vi "string H.vi"() -> ()   [LabVIEW 2020]
panel:
  out "data string":string
  out "*(type *) &x":string
  in  "Numeric":i16
  out "match substring 2":string
  out "before substring 2":string
  out "match substring":string
  out "before substring":string
  out "result string":string
  in  "number":dbl
  in  "age":dbl
  in  "name":string
  out "trimmed length":i32
  out "trimmed string":string
  out "String Subset":string
  out "length":i32
  out "concatonated":string
  in  "String":string
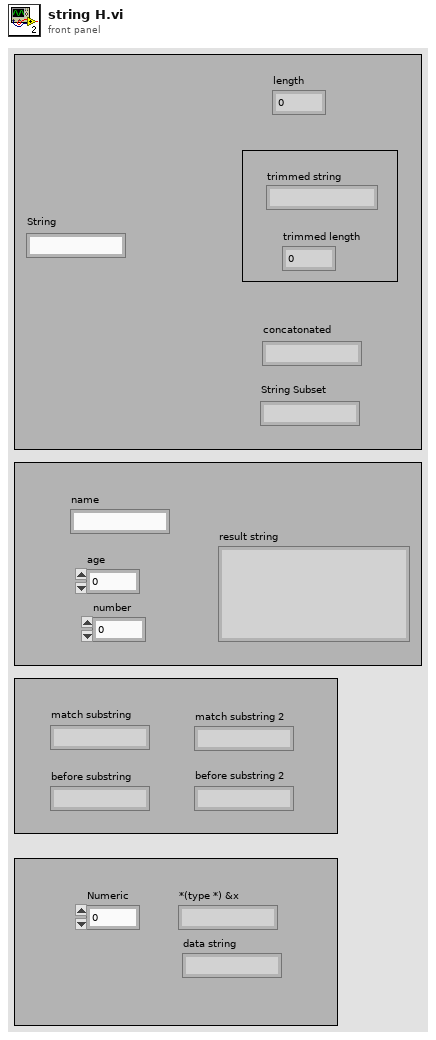
[diagram p1: front panel]
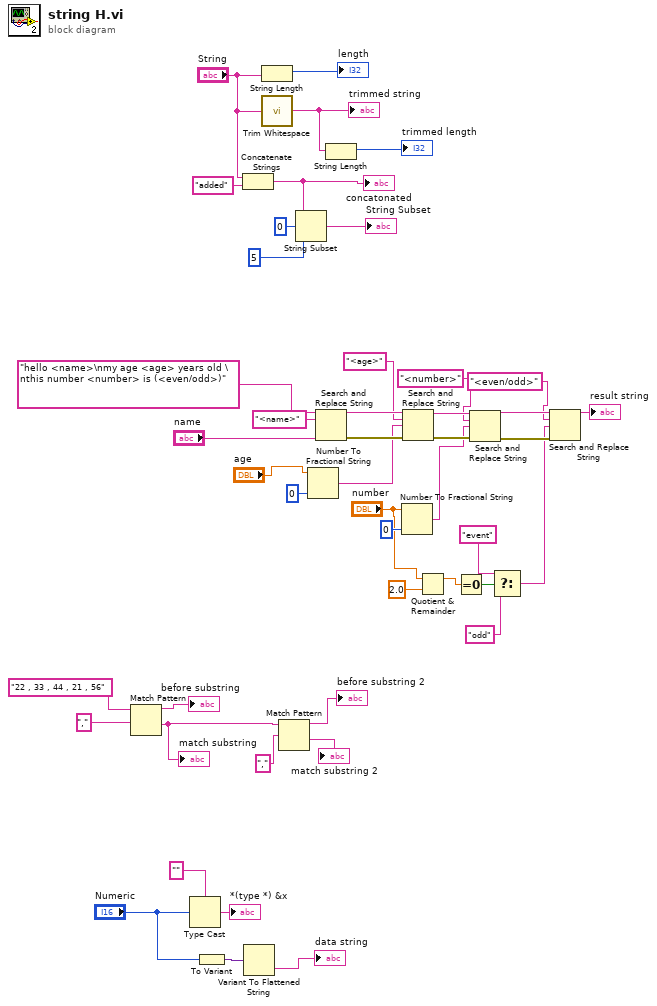
[diagram p0: block diagram]
diagram:
  n1 = Match Pattern(string="22 , 33 , 44 , 21 , 56", regular expression=",") -> (before substring=→"before substring":string, after substring=w6:string)  [unwired: 1 in, 2 out]
  "match substring" <- w6
  n2 = Type Cast(type="", x="Numeric") -> (*(type *) &x=→"*(type *) &x":string)
  n3 = To Variant(anything="Numeric") -> (Variant=w2:variant)
  n4 = Concatenate Strings("String", "added" ("string")) -> (w44:string)
  "concatonated" <- w44
  n5 = Variant To Flattened String(Variant=w2) -> (data string=→"data string":string)  [unwired: 1 out]
  n6 = String Length(string="String") -> (length=→"length":i32)
  n7 = call <vilib>:"Trim Whitespace.vi"("string"="String") -> ("trimmed string"=w38:string)  [unwired: 1 in]
  "trimmed string" <- w38
  n8 = Match Pattern(string=w6, regular expression=",") -> (before substring=→"before substring 2":string, after substring=→"match substring 2":string)  [unwired: 1 in, 2 out]
  n9 = String Subset(string=w44, offset (0)=0, length (rest)=5 ("length (rest)")) -> (substring=→"String Subset":string)
  n10 = Number To Fractional String(number="age", precision (6)=i16 0) -> (F-format string=w29:string)  [unwired: 2 in]
  n11 = Search and Replace String(input string="hello <name>\nmy age <age> years old \nthis number <number> is (<even/odd>)", search string="<name>", replace string="name") -> (result string=w34:string, error out=w33:errorcluster)  [unwired: 5 in, 2 out]
  n12 = String Length(string=w38) -> (length=→"trimmed length":i32)
  n13 = Number To Fractional String(number="number", precision (6)=i16 0) -> (F-format string=w24:string)  [unwired: 2 in]
  n14 = Search and Replace String(input string=w34, search string="<age>", replace string=w29, error in=w33) -> (result string=w27:string, error out=w28:errorcluster)  [unwired: 4 in, 2 out]
  n15 = Quotient & Remainder(x="number", y=2.0) -> (x-y*floor(x/y)=w16:dbl)  [unwired: 1 out]
  n16 = Equal To 0?(x=w16) -> (x = 0?=w15:bool)
  n17 = Search and Replace String(input string=w27, search string="<number>", replace string=w24, error in=w28) -> (result string=w21:string, error out=w20:errorcluster)  [unwired: 4 in, 2 out]
  n18 = Select(t="event" ("search string"), s=w15, f="odd" ("search string")) -> (s? t:f=w14:string)
  n19 = Search and Replace String(input string=w21, search string="<even/odd>", replace string=w14, error in=w20) -> (result string=→"result string":string)  [unwired: 4 in, 3 out]
